vi "Blink - Serial Connection.vi"() -> ()   [LabVIEW 2011, in "LVH-LINX.lvlib"]
doc: "Read one or more analog values from a LINX device using the LINX serial interface."
uses:
  vi.lib/LabVIEW Hacker/LINX/LVH-LINX.lvlib
panel:
  out "LED Value":bool
  in  "Digital Output Channel":u8=13
  in  "Serial Port":refnum<visa-resource-name>
  out "Loop Rate (Hz)":u32
  in  "Stop Button":bool
  # "LINX Device Settings"
  # "LED Value"
  # "Blink (Serial Interface)\n\nThis example demonstrates how to blink and LED on a LINX device connected to \nthe host computer via Serial / USB.\n\nInstructions\n1. Select the COM Port associated with the LINX Device.\n2. Select the Digital Pin connected to the LED.\n3. Click the Run Arrow."
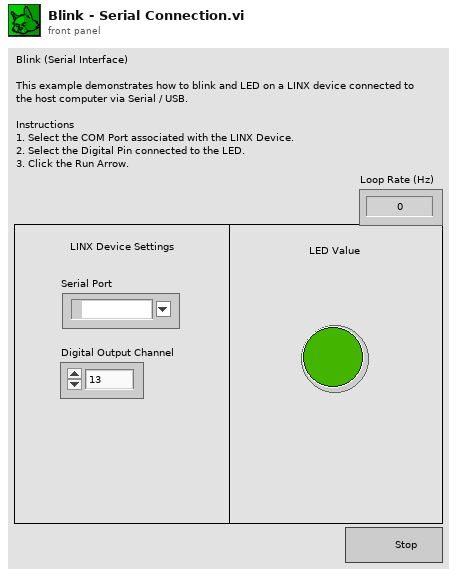
[diagram p1: front panel]
types:
  T1 = typedef "LVH-LINX.lvlib/LINX Ref.ctl" = cluster{"Platform":T2, "Interface":T3, "LINX Device Config":T4}
  T2 = typedef "LVH-LINX.lvlib/Platform.ctl" = enum16{"LINX", "myRIO"}
  T3 = typedef "LVH-LINX.lvlib/Interface.ctl" = enum16{"Serial", "TCP"}
  T4 = typedef "LVH-LINX.lvlib/Device.lvlib/LINX Device Config.ctl" = cluster{"Interface":T3, "COM Port":refnum<visa-resource-name>, "TCP Configuration":T5, "Device Family":T6, "Device ID":u8, "Device Name":string, "TCP Ref":refnum<k5>}
  T5 = typedef "LVH-LINX.lvlib/Device.lvlib/TCP Config.ctl" = cluster{"IP Address":string, "Port":u16}
  T6 = typedef "LVH-LINX.lvlib/Device Family.ctl" = enum8{"National Instruments", "Digilent", "Arduino"}
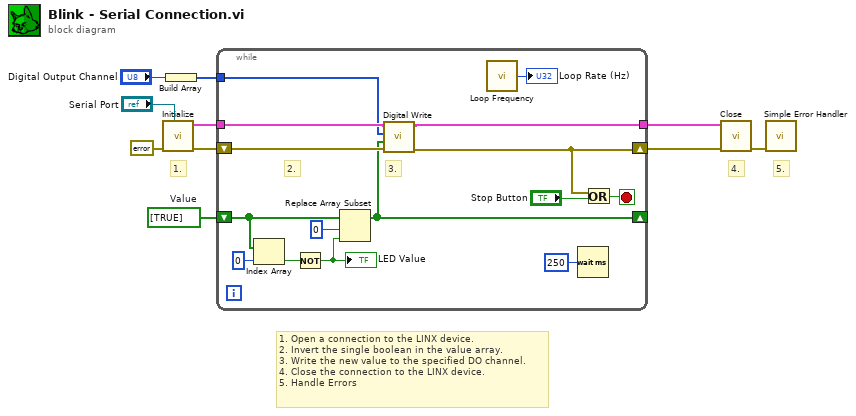
[diagram p0: block diagram]
diagram:
  w1 = bool[] [TRUE]  # Value
  # "1. Open a connection to the LINX device.\n2. Invert the single boolean in the value array.\n3. Write the new value to the specified DO channel.\n4. Close the connection to the LINX device.\n5. Handle Errors"
  # "5."
  # "4."
  # "1."
  n1 = call "Initialize.vi"("Serial Port"="Serial Port", "Error In"=errorcluster {"status"=FALSE, "code"=0, "source"=""}) -> ("Error Out"=w9:errorcluster, "LINX Ref"=w10:T1)  [unwired: 7 in, 1 out]
  n2 = Build Array("Digital Output Channel") -> (w2:u8[])
  n3 = while {
    tunnel: w10 -> [w22]
    tunnel: [w21] -> w8
    shift-right: [w19] -> w7
    shift-left: w9 -> [w20]
    tunnel: w2 -> [w18]
    shift-right: [w12] -> _
    shift-left: w1 -> [w17]
    stop <- w25 stop-if-true
    # "2."
    # "3."
    n4 = Index Array(array=w17, index=0) -> (element=w15:bool)
    n5 = Not(x=w15) -> (.not. x?=w14:bool)
    "LED Value" <- w14
    n6 = Replace Array Subset(array=w17, new element=w14, index=0) -> (w12:bool[])
    n7 = call "Digital Write.vi"("Error In"=w20, "Values"=w12, "Channels"=w18, "LINX Resource"=w22) -> ("Error Out"=w19:errorcluster, "LINX Resource"=w21:T1)  [unwired: 6 in]
    n8 = call "Loop Frequency.vi"() -> ("Loop Rate (Hz)"=→"Loop Rate (Hz)":u32)
    n9 = Wait (ms)(milliseconds to wait=u32 250) -> ()  [unwired: 1 out]
    n10 = Or(x=w19, y="Stop Button") -> (x .or. y?=w25:bool)
  }
  n11 = call "Close.vi"("Error In"=w7, "LINX Resource"=w8) -> ("Error Out"=w5:errorcluster)  [unwired: 8 in, 1 out]
  n12 = call <vilib>:"Simple Error Handler.vi"("error in (no error)"=w5) -> ()  [unwired: 4 in, 5 out]
